vi "Unflatten UIP Value.vi"(10 "String Value":string, 11 "UIP In":refnum<class "TemplateUIP.lvclass">) -> (0 "Error Out":errorcluster, 3 "UIP Out":refnum<class "TemplateUIP.lvclass">)   [LabVIEW 2020, in "UIM.lvlib" / "TemplateUIP.lvclass"]
uses:
  TemplateUIP.lvclass
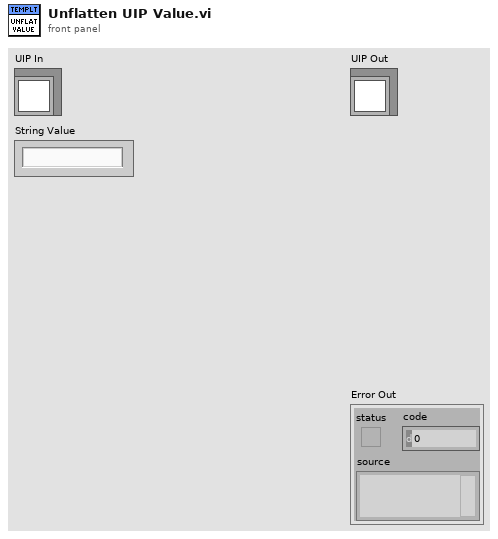
[diagram p1: front panel]
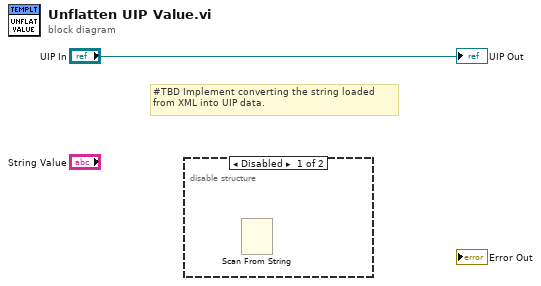
[diagram p0: block diagram]
diagram:
  # "#TBD Implement converting the string loaded\nfrom XML into UIP data."
  n1 = disable-structure shown="Disabled" {
    frame Disabled {
      n2 = Scan From String "Scan From String"() -> ()  [unwired: 6 in, 3 out]
    }
    frame Enabled {
    }
  }
  "UIP Out" <- "UIP In"
